vi "Tektronix AFG 1000 Series Generate Arbitrary Waveform.vi"() -> ()   [LabVIEW 2016]
doc: "Demonstrates how to configure then create an arbitrary waveform."
uses:
  <instrlib>/Tektronix AFG 1000 Series/Tektronix AFG 1000 Series.lvlib
panel:
  in  "Phase Unit (0: Radian)":u16(ring) items=["Radians", "Degrees"]
  in  "Phase (0)":dbl
  in  "Channel (1: Channel 1)":u16(ring)=1 items=["Channel 1"=1, "Channel 2"=2]
  in  "Enable Output (T: Enable)":bool=TRUE
  in  "Frequency (1000 Hz)":dbl=1000.0
  in  "DC Offset (0 V)":dbl
  in  "Gain (1 V)":dbl=1.0
  in  "Arbitrary Waveform Data":dbl[](array[numeric])=[1.0, 2.0, -1.0, 0.0, -2.0]
  in  "VISA resource name":refnum<visa-resource-name>
  # "(c) 2016 National Instruments.  ALL RIGHTS RESERVED."
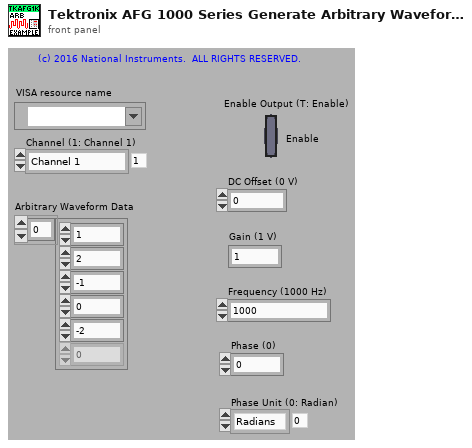
[diagram p1: front panel]
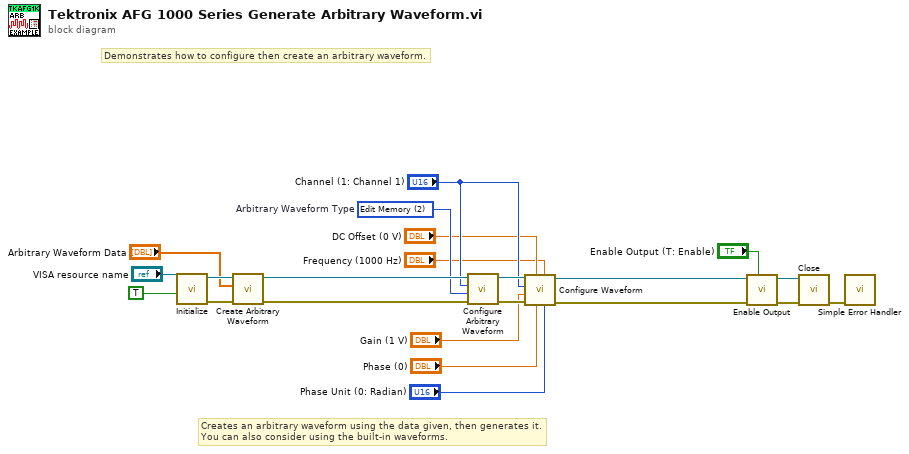
[diagram p0: block diagram]
diagram:
  w11 = u16 2 items=["Built-in", "User Waveform", "Edit Memory", "EFile"]  # Arbitrary Waveform Type
  # "Demonstrates how to configure then create an arbitrary waveform."
  # "Creates an arbitrary waveform using the data given, then generates it.\nYou can also consider using the built-in waveforms."
  n1 = call <instrlib>:"Initialize.vi"("Reset (True)"=TRUE, "VISA resource name"="VISA resource name") -> ("error out"=w21:errorcluster, "VISA resource name out"=w19:refnum<visa-resource-name>)  [unwired: 8 in]
  n2 = call <instrlib>:"Create Arbitrary Waveform.vi"("error in (no error)"=w21, "Arbitrary Waveform Data"="Arbitrary Waveform Data", "VISA resource name"=w19) -> ("error out"=w15:errorcluster, "VISA resource name out"=w16:refnum<visa-resource-name>)  [unwired: 7 in]
  n3 = call <instrlib>:"Configure Arbitrary Waveform.vi"("error in (no error)"=w15, "Arbitrary Waveform Type (0: Built-in)"=w11, "Channel (1: Channel 1)"="Channel (1: Channel 1)", "VISA resource name"=w16) -> ("error out"=w10:errorcluster, "VISA resource name out"=w8:refnum<visa-resource-name>)  [unwired: 6 in]
  n4 = call <instrlib>:"Configure Waveform.vi"("Phase Unit (0: Radian)"="Phase Unit (0: Radian)", "Frequency (1000 Hz)"="Frequency (1000 Hz)", "Phase (0)"="Phase (0)", "DC Offset (0.00 V)"="DC Offset (0 V)", "error in (no error)"=w10, "Amplitude (1 Vpp)"="Gain (1 V)", "Channel (1 Channel 1)"="Channel (1: Channel 1)", "VISA resource name"=w8) -> ("error out"=w9:errorcluster, "VISA resource name out"=w7:refnum<visa-resource-name>)  [unwired: 2 in]
  n5 = call <instrlib>:"Enable Output.vi"("Enable Output (T: Enable)"="Enable Output (T: Enable)", "error in (no error)"=w9, "VISA resource name"=w7) -> ("error out"=w12:errorcluster, "VISA resource name out"=w13:refnum<visa-resource-name>)  [unwired: 7 in]
  n6 = call <instrlib>:"Close.vi"("error in (no error)"=w12, "VISA resource name"=w13) -> ("error out"=w22:errorcluster)  [unwired: 9 in]
  n7 = call <vilib>:"Simple Error Handler.vi"("error in (no error)"=w22) -> ()  [unwired: 4 in, 5 out]
